vi "laneleftright413.vi"() -> ()   [LabVIEW 2015]
uses:
  <vilib>/Analysis/1siggen.llb/Ramp Pattern by Samples.vi
  G_SEN.vi
  <vilib>/Analysis/1siggen.llb/Ramp Pattern by Delta.vi
  G_ALL.vi
  G_LCM.vi
  <vilib>/Analysis/polynomials.llb/1D Polynomial Evaluation (DBL).vi
  <vilib>/Analysis/NI_AALBase.lvlib
  <vilib>/Analysis/NI_AALPro.lvlib
panel:
  out "lnum":dbl format="%.2f"
  out "rnum":dbl format="%.2f"
  out "Waveform Graph 2":dbl[](graph)
  out "w0":dbl[](array[numeric])
  out "y0":dbl[](array[numeric])
  out "x0":dbl[](array[numeric])
  out "Waveform Graph":dbl[](graph)
  out "Coeff left":dbl[](array[numeric])
  in  "iter":i32
  out "Coeff right":dbl[](array[numeric])
  out "XY Graph 4":cluster{"Y":dbl[], "Y":dbl[]}[](graph)=[{"Y"=array[3210 elements], "Y"=array[3210 elements]}, {"Y"=[-0.0, 0.001154394197769193, 0.004617650635850623, 0.010389990872226917, 0.018471784248973222, 0.02886354801042046, 0.041565947468740205, 0.056579796217107514, 0.0739060563904701, 0.0935458389742223, 0.11550040416098284, 0.13977116175580306, 0.16635967162997645, 0.19526764422393228, 0.2264969410994837, 0.26004957554195585, 0.2959277132125635, 0.3341336728515216, 0.374669927032528, 0.417539102969144, 0.4627439833735707, 0.5102875073687159, 0.560172771454063, 0.6124030305261954, 0.6669816989546717, 0.7239123517142048, 0.7831987255740245, 0.8448447203451934, 0.9088544001870815, 0.975231994973953, 1.0439819017227023, 1.1151086860829622, 1.1886170838907617, 1.2645120027869723, 1.342798523901962, 1.42348190360768, 1.5065675753387922, 1.592061151484188, 1.6799684253507792, 1.770295373200753, 1.8630481563645134, 1.9582331234307588, 2.0558568125157564, 2.1559259536137603, 2.258447471030621], "Y"=[0.0, 0.5, 1.0, 1.5, 2.0, 2.5, 3.0, 3.5, 4.0, 4.5, 5.0, 5.5, 6.0, 6.5, 7.0, 7.5, 8.0, 8.5, 9.0, 9.5, 10.0, 10.5, 11.0, 11.5, 12.0, 12.5, 13.0, 13.5, 14.0, 14.5, 15.0, 15.5, 16.0, 16.5, 17.0, 17.5, 18.0, 18.5, 19.0, 19.5, 20.0, 20.5, 21.0, 21.5, 22.0]}, {"Y"=[0.362252581831572], "Y"=[-0.8199241909738847]}, {"Y"=array[210 elements], "Y"=array[210 elements]}, {"Y"=[-0.925, -0.925, -0.925, -0.6775, -0.6775, -0.925, -0.925, -0.925, -0.925, -0.6775, -0.6775, -0.925, -0.925, -0.925, 0.9025, 0.9025, 0.9025, 0.6775, 0.6775, 0.9025, 0.9025, 0.9025, 0.9025, 0.6775, 0.6775, 0.9025, 0.9025, 0.9025, -0.925], "Y"=[-0.75, -0.224, 0.224, 0.224, -0.224, -0.224, 0.224, 2.415, 2.885, 2.885, 2.415, 2.415, 2.885, 3.5, 3.5, 2.885, 2.415, 2.415, 2.885, 2.885, 2.415, 0.224, -0.224, -0.224, 0.224, 0.224, -0.224, -0.75, -0.75]}, {"Y"=[0.171875, 0.15377271904051304, 0.1346290179491043, 0.11445423440635205, 0.09325870609283447, 0.07105277068912982, 0.04784676587581635, 0.02365102933347224, -0.0015241012573242174, -0.02766828821599482, -0.05477119386196136, -0.08282248051464558, -0.11181181049346922, -0.14172884611785413, -0.17256324970722198, -0.20430468358099463, -0.23694281005859374, -0.27046729145944115, -0.30486779010295867, -0.340133968308568, -0.3762554883956909, -0.41322201268374914, -0.4510232034921646, -0.4896487231403589], "Y"=[0.0, 0.5, 1.0, 1.5, 2.0, 2.5, 3.0, 3.5, 4.0, 4.5, 5.0, 5.5, 6.0, 6.5, 7.0, 7.5, 8.0, 8.5, 9.0, 9.5, 10.0, 10.5, 11.0, 11.5]}, {"Y"=[1.796875, 1.778772719040513, 1.7596290179491043, 1.739454234406352, 1.7182587060928345, 1.6960527706891297, 1.6728467658758164, 1.6486510293334722, 1.6234758987426758, 1.5973317117840051, 1.5702288061380387, 1.5421775194853544, 1.513188189506531, 1.483271153882146, 1.452436750292778, 1.4206953164190055, 1.3880571899414063, 1.354532708540559, 1.3201322098970414, 1.284866031691432, 1.248744511604309, 1.2117779873162509, 1.1739767965078354, 1.135351276859641, 1.0959117660522462, 1.0556686017662287, 1.014632121682167, 0.9728126634806396, 0.9302205648422242, 0.8868661634474992], "Y"=[0.0, 0.5, 1.0, 1.5, 2.0, 2.5, 3.0, 3.5, 4.0, 4.5, 5.0, 5.5, 6.0, 6.5, 7.0, 7.5, 8.0, 8.5, 9.0, 9.5, 10.0, 10.5, 11.0, 11.5, 12.0, 12.5, 13.0, 13.5, 14.0, 14.5]}, {"Y"=[-1.453125, -1.471227280959487, -1.4903709820508957, -1.510545765593648, -1.5317412939071655, -1.5539472293108703, -1.5771532341241836, -1.6013489706665278, -1.6265241012573242, -1.6526682882159949, -1.6797711938619613, -1.7078224805146456, -1.736811810493469, -1.766728846117854, -1.797563249707222, -1.8293046835809945, -1.8619428100585937, -1.895467291459441, -1.9298677901029586], "Y"=[0.0, 0.5, 1.0, 1.5, 2.0, 2.5, 3.0, 3.5, 4.0, 4.5, 5.0, 5.5, 6.0, 6.5, 7.0, 7.5, 8.0, 8.5, 9.0]}, {"Y"=[0.171875, 0.2568230007600336, 0.3384052130063493, 0.44574342526006827, 0.5205081969556753, 0.5917680690742042, 0.659409530134929, 0.7229937549325056, 0.7835496148685115, 0.8405449546633443, 0.9258576868463875], "Y"=[-20.239964538708662, -19.725637940364884, -19.211158961966362, -18.6998967366845, -18.19022720070031, -17.681887266143153, -17.17615515566314, -16.67683575591291, -16.176265245349786, -15.679082775270938, -15.183754484614711]}, {"Y"=[7.134647485270904], "Y"=[38.71960961082238]}, {"Y"=array[980 elements], "Y"=array[980 elements]}, {"Y"=[], "Y"=[]}]
  out "w":dbl[](array[numeric])
  out "y":dbl[](array[numeric])
  out "x":dbl[](array[numeric])
  out "gap":dbl
  out "rin":dbl[](array[numeric])
  out "rout":dbl[](array[numeric])
  out "r":dbl[](array[numeric])
  out "wgain":dbl[](array[numeric])
  out "y_end":dbl[](array[numeric])=[0.8601491478953653, 0.8717844136967624, 0.882947592858927, 0.8936326403234123, 0.9038337699485205, 0.9135454576426009, 0.9227624443554423, 0.9314797389261423, 0.9396926207859084, 0.9473966425143293, 0.9545876322477319, 0.9612616959383189, 0.9674152194628639, 0.9730448705798238, 0.9781476007338057, 0.9827206467064133, 0.9867615321125792, 0.9902680687415704, 0.993238357741943, 0.9956707906498045, 0.9975640502598242, 0.9989171113385246, 0.9997292411794617, 1.0, 0.9997292411794617, 0.9989171113385246, 0.9975640502598242, 0.9956707906498045, 0.993238357741943, 0.9902680687415704, 0.9867615321125792, 0.9827206467064133]
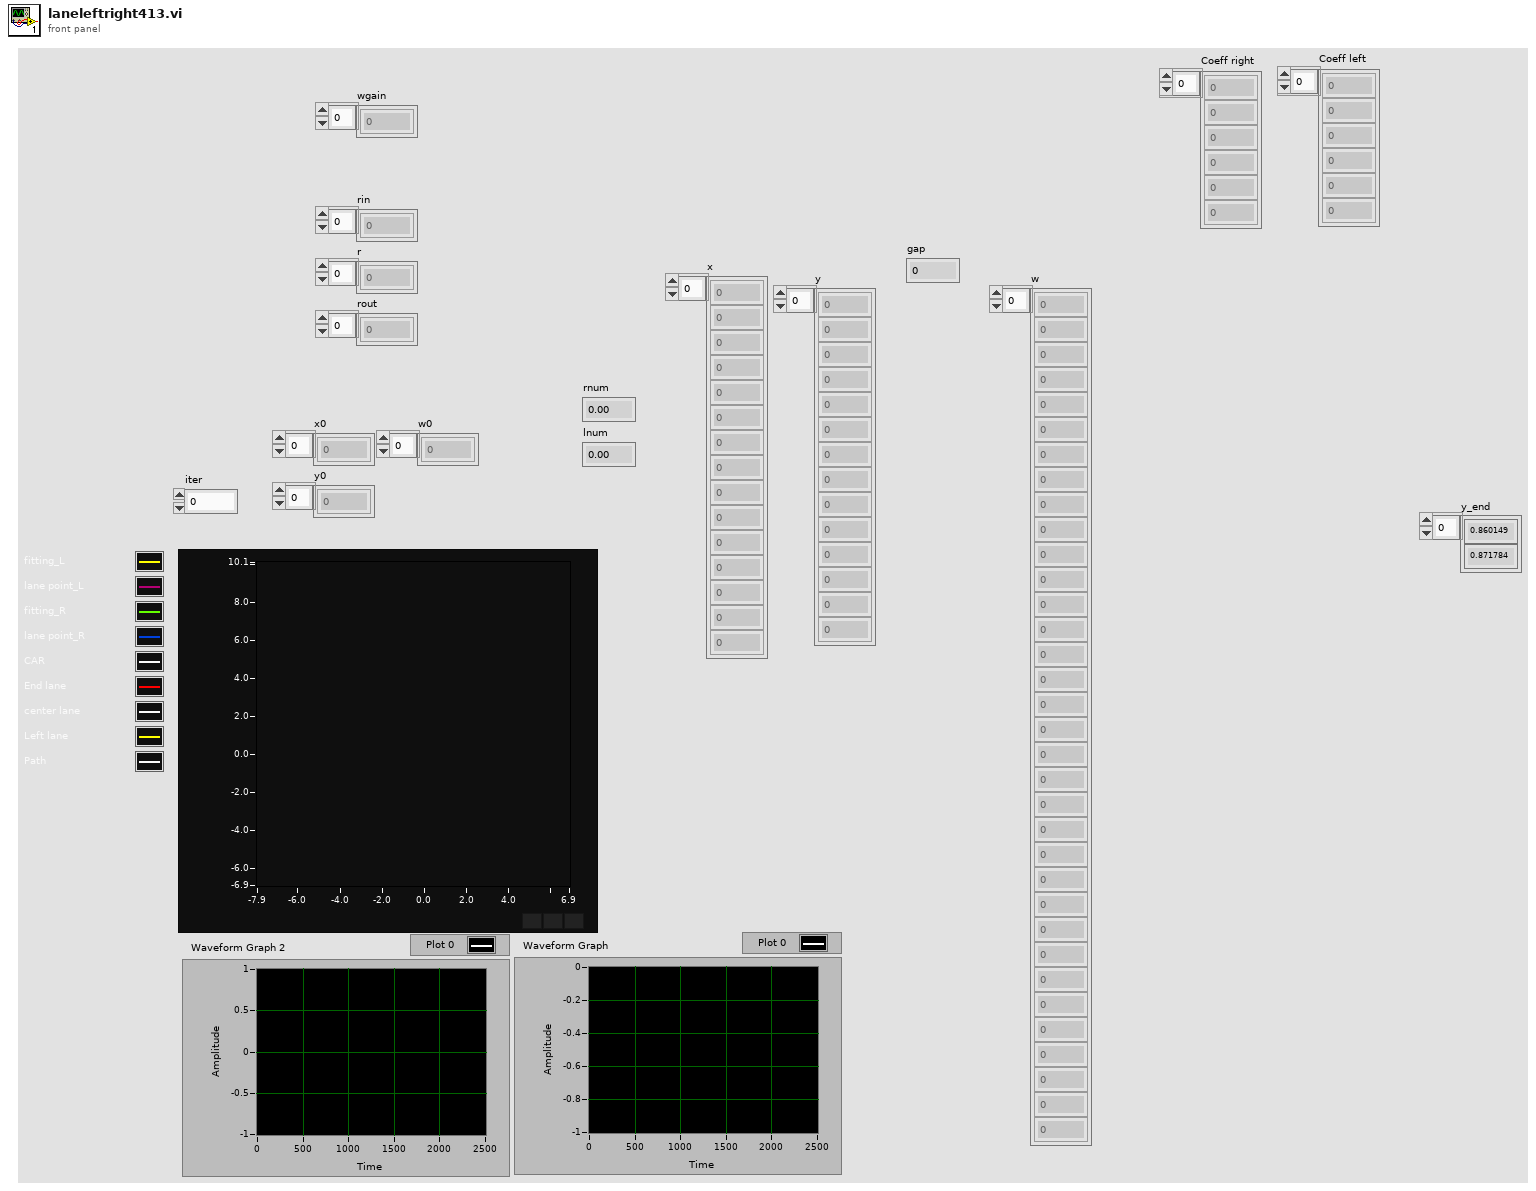
[diagram p1: front panel]
types:
  T1 = cluster{"C_Wheel base":dbl, "ratio_steer":dbl, "Overall width":dbl, "af":dbl, "turn radius":dbl, "eval":dbl, "ap":dbl, "an":dbl, "Vmax":dbl, "mu":dbl, "Vlast":dbl}
  T2 = cluster{"hash":i64, "sys time":i64, "size":i64, "x":dbl[], "y":dbl[], "point_flag":i32[]}
  T3 = cluster{"Numeric":bool, "Numeric":i32, "Rotational position":dbl, "Rotational position":dbl}[]
  T4 = cluster{bool, "Rotational position":dbl, "Rotational position":dbl}[]
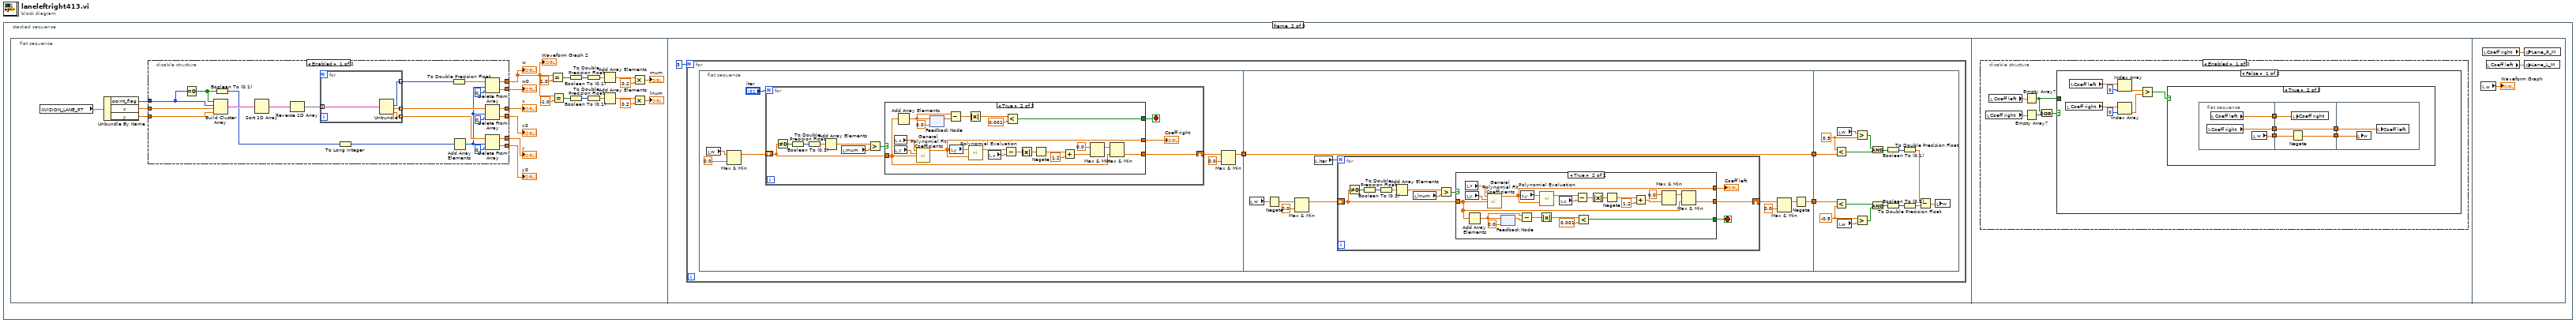
[diagram p0: block diagram]
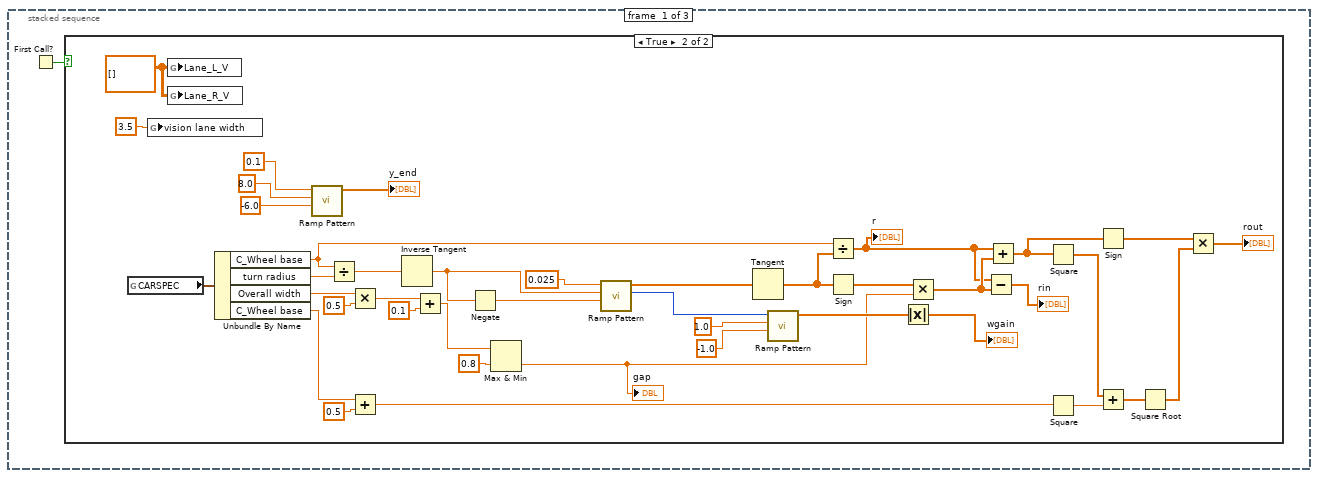
[diagram p2: hidden frame]
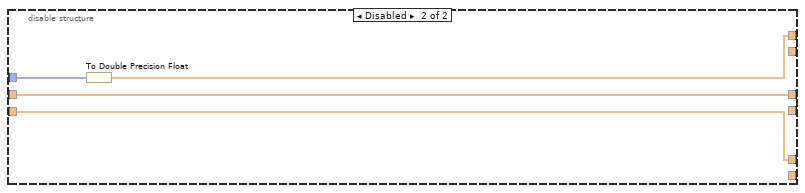
[diagram p4: hidden frame]
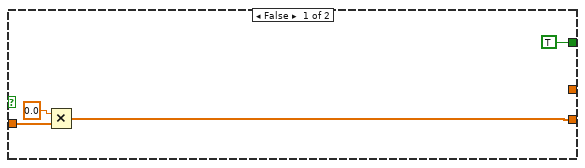
[diagram p5: hidden frame]
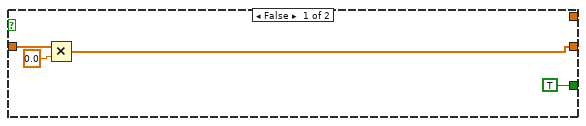
[diagram p6: hidden frame]
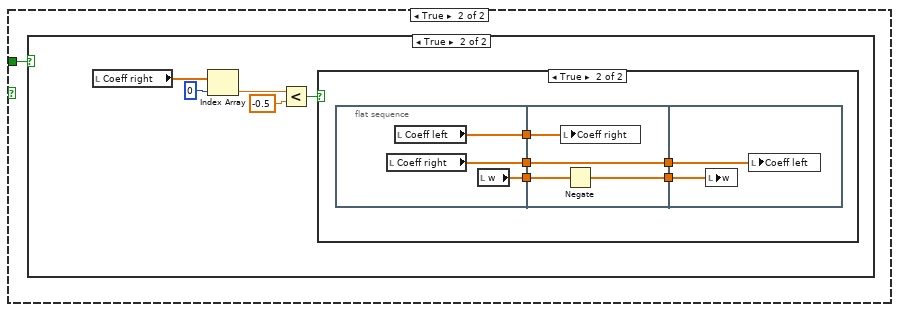
[diagram p8: hidden frame]
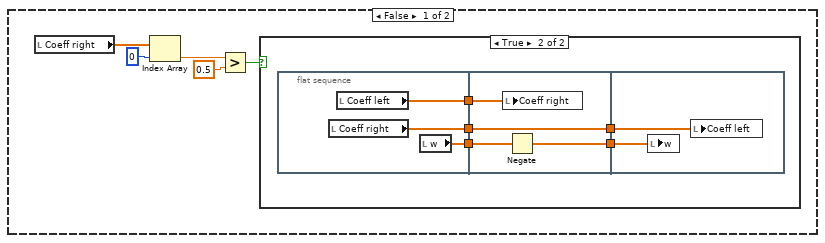
[diagram p9: hidden frame]
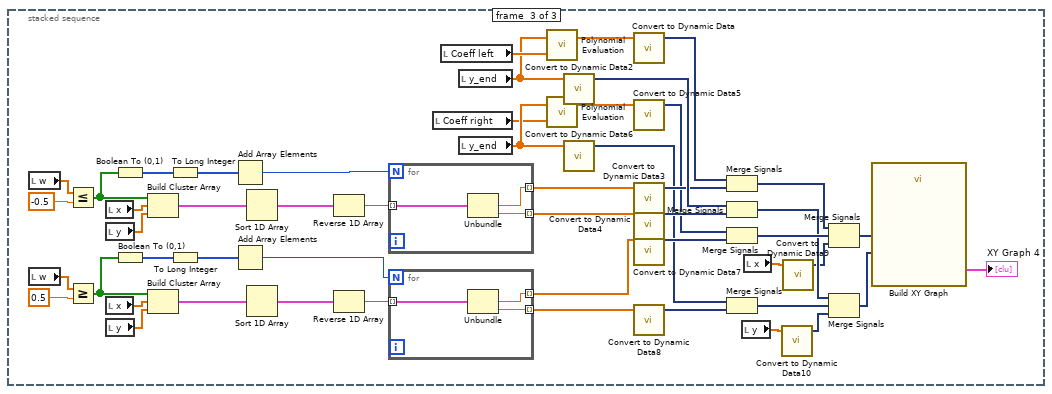
[diagram p13: hidden frame]
diagram:
  n1 = stacked-sequence {
    frame #0 {
      n2 = First Call?() -> (First Call?: T/F=w1:bool)
      n3 = case shown="True" w1 {
        frame False {
        }
        frame True {
          w37 = dbl[][] [] ("Lane_R_V")
          n4 = global read "G_ALL.vi" "CARSPEC"() -> (w10:T1)
          n5 = global write "G_SEN.vi" "vision lane width"(3.5 ("vision lane width")) -> ()
          n6 = global write "G_SEN.vi" "Lane_L_V"(w37) -> ()
          n7 = global write "G_SEN.vi" "Lane_R_V"(w37) -> ()
          n8 = Unbundle By Name(w10) -> ("C_Wheel base"=w17:dbl, "turn radius"=w11:dbl, "Overall width"=w18:dbl, "C_Wheel base"=w3:dbl)
          n9 = call-poly <vilib>:"Ramp Pattern.vi"("start"=-6.0, "end"=8.0, "delta"=0.1) -> ("Ramp Pattern"=→"y_end":dbl[])  [unwired: 6 in, 2 out]
          n10 = Divide(x=w17, y=w11) -> (x/y=w12:dbl)
          n11 = Multiply(x=w18, y=0.5) -> (x*y=w9:dbl)
          n12 = Add(x=w3, y=0.5) -> (x+y=w2:dbl)
          n13 = Inverse Tangent(1:w12) -> (0:w14:dbl)
          n14 = Add(x=w9, y=0.1) -> (x+y=w6:dbl)
          n15 = Negate(x=w14) -> (-x=w13:dbl)
          n16 = Max & Min(x=w6, y=0.8) -> (min(x,y)=w5:dbl)  [unwired: 1 out]
          "gap" <- w5
          n17 = call-poly <vilib>:"Ramp Pattern.vi"("start"=w13, "end"=w14, "delta"=0.025) -> ("samples"=w32:i32, "Ramp Pattern"=w16:dbl[])  [unwired: 6 in, 1 out]
          n18 = Tangent(1:w16) -> (0:w20:dbl[])
          n19 = call-poly <vilib>:"Ramp Pattern.vi"("start"=-1.0, "end"=1.0, "samples"=w32) -> ("Ramp Pattern"=w35:dbl[])  [unwired: 7 in, 1 out]
          n20 = Divide(x=w17, y=w20) -> (x/y=w23:dbl[])
          "r" <- w23
          n21 = Sign(1:w20) -> (0:w21:dbl[])
          n22 = Absolute Value(x=w35) -> (abs(x)=→"wgain":dbl[])
          n23 = Multiply(x=w21, y=w5) -> (x*y=w24:dbl[])
          n24 = Subtract(x=w23, y=w24) -> (x-y=→"rin":dbl[])
          n25 = Add(x=w23, y=w24) -> (x+y=w28:dbl[])
          n26 = Square(x=w28) -> (x^2=w25:dbl[])
          n27 = Square(x=w2) -> (x^2=w26:dbl)
          n28 = Sign(1:w28) -> (0:w30:dbl[])
          n29 = Add(x=w25, y=w26) -> (x+y=w27:dbl[])
          n30 = Square Root(x=w27) -> (sqrt(x)=w29:dbl[])
          n31 = Multiply(x=w30, y=w29) -> (x*y=→"rout":dbl[])
        }
      }
    }
    frame #1 {
      n32 = flat-sequence {
        frame #0 {
          n33 = global read "G_LCM.vi" "VISION_LANE_PT"() -> (w66:T2)
          n34 = Unbundle By Name(w66) -> ("point_flag"=w58:i32[], "x"=w65:dbl[], "y"=w64:dbl[])
          n35 = disable-structure shown="Enabled" {
            disable-tunnel: w58 -> [w67 w94]
            disable-tunnel: w65 -> [w68 w95]
            disable-tunnel: w64 -> [w69 w96]
            disable-tunnel: [w81 _] -> w63
            disable-tunnel: [w80 w95] -> w62
            disable-tunnel: [w77 _] -> w61
            disable-tunnel: [w76 w96] -> w60
            disable-tunnel: [w71 _] -> w59
            disable-tunnel: [w70 w97] -> w49
            frame Enabled {
              n36 = Equal To 0?(x=w67) -> (x = 0?=w84:bool[])
              n37 = Build Cluster Array(w84, w67, w68, w69) -> (w89:T3)
              n38 = Boolean To (0,1)(Boolean=w84) -> (0, 1=w83:i16[])
              n39 = Sort 1D Array(array=w89) -> (sorted array=w87:T3)
              n40 = Reverse 1D Array(array=w87) -> (reversed array=w86:T3)
              n41 = for {
                tunnel: w86 -> [w93] mode=indexing
                tunnel: [w92] -> w88 mode=indexing
                tunnel: [w91] -> w78 mode=indexing
                tunnel: [w90] -> w73 mode=indexing
                n42 = Unbundle(w93) -> ("Numeric"=w90:i32, "Rotational position"=w92:dbl, "Rotational position"=w91:dbl)  [unwired: 1 out]
              }
              n43 = To Long Integer(number=w83) -> (32bit integer=w82:i32[])
              n44 = To Double Precision Float(number=w73) -> (double precision float=w72:dbl[])
              n45 = Add Array Elements(numeric array=w82) -> (sum=w74:i32)
              n46 = Delete From Array(array=w72, length=w74, index=0) -> (deleted portion=w71:dbl[], array with subset deleted=w70:dbl[])
              n47 = Delete From Array(array=w88, length=w74, index=0) -> (deleted portion=w81:dbl[], array with subset deleted=w80:dbl[])
              n48 = Delete From Array(array=w78, length=w74, index=0) -> (deleted portion=w77:dbl[], array with subset deleted=w76:dbl[])
            }
            frame Disabled {
              n49 = To Double Precision Float(number=w94) -> (double precision float=w97:dbl[])
            }
          }
          "x" <- w62
          "y" <- w60
          "w" <- w49
          "x0" <- w63
          "y0" <- w61
          "w0" <- w59
          "Waveform Graph 2" <- w49
          n50 = Equal?(x=w49, y=1.0) -> (x = y?=w54:bool[])
          n51 = Equal?(x=w49, y=-1.0) -> (x = y?=w53:bool[])
          n52 = Boolean To (0,1)(Boolean=w54) -> (0, 1=w56:i16[])
          n53 = Boolean To (0,1)(Boolean=w53) -> (0, 1=w51:i16[])
          n54 = To Double Precision Float(number=w56) -> (double precision float=w55:dbl[])
          n55 = To Double Precision Float(number=w51) -> (double precision float=w52:dbl[])
          n56 = Add Array Elements(numeric array=w55) -> (sum=w48:dbl)
          n57 = Add Array Elements(numeric array=w52) -> (sum=w44:dbl)
          n58 = Multiply(x=w48, y=0.2) -> (x*y=→"rnum":dbl)
          n59 = Multiply(x=w44, y=0.2) -> (x*y=→"lnum":dbl)
        }
        frame #1 {
          n60 = for {
            N: 3 -> [_]
            n61 = flat-sequence {
              tunnel: [w105] -> w100
              tunnel: [w149] -> w101
              tunnel: w100 -> [w149]
              tunnel: [w148] -> w99
              tunnel: w101 -> [w202]
              tunnel: w99 -> [w198]
              frame #0 {
                n62 = local read "w"() -> (w103:dbl[])
                n63 = Max & Min(x=w103, y=0.0) -> (max(x,y)=w102:dbl[])  [unwired: 1 out]
                n64 = for {
                  N: "iter" -> [_]
                  shift-right: [w116] -> w108
                  shift-left: w102 -> [w115]
                  stop <- w118 stop-if-true
                  n65 = Not Equal To 0?(x=w115) -> (x != 0?=w114:bool[])
                  n66 = Boolean To (0,1)(Boolean=w114) -> (0, 1=w113:i16[])
                  n67 = To Double Precision Float(number=w113) -> (double precision float=w112:dbl[])
                  n68 = Add Array Elements(numeric array=w112) -> (sum=w111:dbl)
                  n69 = local read "rnum"() -> (w109:dbl)
                  n70 = Greater?(x=w111, y=w109) -> (0:w110:bool)
                  n71 = case shown="True" w110 {
                    tunnel: [TRUE w129] -> w118
                    tunnel: [_ w128] -> w117
                    tunnel: [w119 w127] -> w116
                    tunnel: w115 -> [w121 w123]
                    frame False {
                      n72 = Multiply(x=0.0, y=w121) -> (x*y=w119:dbl[])
                    }
                    frame True {
                      n73 = local read "x"() -> (w144:dbl[])
                      n74 = local read "y"() -> (w143:dbl[])
                      n75 = Add Array Elements(numeric array=w123) -> (sum=w134:dbl)
                      n76 = call <vilib>:"General Polynomial Fit Coefficients.vi"("Y"=w144, "X"=w143, "Weight"=w123) -> ("Polynomial Coefficients"=w128:dbl[])  [unwired: 11 in, 1 out]
                      n77 = feedback #1(0.0) -> (w135:dbl)
                      n78 = feedback-in #1(w134) -> ()
                      n79 = Subtract(x=w134, y=w135) -> (x-y=w132:dbl)
                      n80 = local read "y"() -> (w136:dbl[])
                      n81 = Absolute Value(x=w132) -> (abs(x)=w131:dbl)
                      n82 = call-poly <vilib>:"Polynomial Evaluation.vi"("P(x)"=w128, "A"=w136) -> ("P(A)"=w137:dbl[])  [unwired: 1 out]
                      n83 = local read "x"() -> (w138:dbl[])
                      n84 = Subtract(x=w137, y=w138) -> (x-y=w139:dbl[])
                      n85 = Less?(x=w131, y=0.001) -> (x < y?=w129:bool)
                      n86 = Absolute Value(x=w139) -> (abs(x)=w140:dbl[])
                      n87 = Negate(x=w140) -> (-x=w141:dbl[])
                      n88 = Add(x=w141, y=1.2) -> (x+y=w126:dbl[])
                      n89 = Max & Min(x=0.0, y=w126) -> (max(x,y)=w124:dbl[])  [unwired: 1 out]
                      n90 = Max & Min(x=w124, y=w123) -> (min(x,y)=w127:dbl[])  [unwired: 1 out]
                    }
                  }
                  "Coeff right" <- w117
                }
                n91 = Max & Min(x=w108, y=0.0) -> (max(x,y)=w105:dbl[])  [unwired: 1 out]
              }
              frame #1 {
                n92 = local read "w"() -> (w151:dbl[])
                n93 = Negate(x=w151) -> (-x=w146:dbl[])
                n94 = Max & Min(x=w146, y=0.0) -> (max(x,y)=w145:dbl[])  [unwired: 1 out]
                n95 = local read "iter"() -> (w150:i32)
                n96 = for {
                  N: w150 -> [_]
                  shift-right: [w162] -> w153
                  shift-left: w145 -> [w157]
                  stop <- w163 stop-if-true
                  n97 = Not Equal To 0?(x=w157) -> (x != 0?=w158:bool[])
                  n98 = Boolean To (0,1)(Boolean=w158) -> (0, 1=w159:i16[])
                  n99 = To Double Precision Float(number=w159) -> (double precision float=w160:dbl[])
                  n100 = Add Array Elements(numeric array=w160) -> (sum=w161:dbl)
                  n101 = local read "lnum"() -> (w155:dbl)
                  n102 = Greater?(x=w161, y=w155) -> (0:w156:bool)
                  n103 = case shown="True" w156 {
                    tunnel: [_ w181] -> w164
                    tunnel: [TRUE w174] -> w163
                    tunnel: w157 -> [w167 w170]
                    tunnel: [w166 w169] -> w162
                    frame False {
                      n104 = Multiply(x=w167, y=0.0) -> (x*y=w166:dbl[])
                    }
                    frame True {
                      n105 = local read "x"() -> (w190:dbl[])
                      n106 = local read "y"() -> (w189:dbl[])
                      n107 = Add Array Elements(numeric array=w170) -> (sum=w179:dbl)
                      n108 = call <vilib>:"General Polynomial Fit Coefficients.vi"("Y"=w190, "X"=w189, "Weight"=w170) -> ("Polynomial Coefficients"=w181:dbl[])  [unwired: 11 in, 1 out]
                      n109 = feedback #2(0.0) -> (w180:dbl)
                      n110 = feedback-in #2(w179) -> ()
                      n111 = Subtract(x=w179, y=w180) -> (x-y=w177:dbl)
                      n112 = local read "y"() -> (w182:dbl[])
                      n113 = Absolute Value(x=w177) -> (abs(x)=w176:dbl)
                      n114 = call-poly <vilib>:"Polynomial Evaluation.vi"("P(x)"=w181, "A"=w182) -> ("P(A)"=w183:dbl[])  [unwired: 1 out]
                      n115 = local read "x"() -> (w184:dbl[])
                      n116 = Subtract(x=w183, y=w184) -> (x-y=w185:dbl[])
                      n117 = Less?(x=w176, y=0.001) -> (x < y?=w174:bool)
                      n118 = Absolute Value(x=w185) -> (abs(x)=w186:dbl[])
                      n119 = Negate(x=w186) -> (-x=w187:dbl[])
                      n120 = Add(x=w187, y=1.2) -> (x+y=w171:dbl[])
                      n121 = Max & Min(x=0.0, y=w171) -> (max(x,y)=w173:dbl[])  [unwired: 1 out]
                      n122 = Max & Min(x=w173, y=w170) -> (min(x,y)=w169:dbl[])  [unwired: 1 out]
                    }
                  }
                  "Coeff left" <- w164
                }
                n123 = Max & Min(x=w153, y=0.0) -> (max(x,y)=w154:dbl[])  [unwired: 1 out]
                n124 = Negate(x=w154) -> (-x=w148:dbl[])
              }
              frame #2 {
                w199 = -0.5
                w201 = 0.5
                n125 = Less?(x=w201, y=w202) -> (x < y?=w205:bool[])
                n126 = Less?(x=w198, y=w199) -> (x < y?=w203:bool[])
                n127 = local read "w"() -> (w207:dbl[])
                n128 = local read "w"() -> (w200:dbl[])
                n129 = Greater?(x=w207, y=w201) -> (0:w206:bool[])
                n130 = Greater?(x=w199, y=w200) -> (0:w204:bool[])
                n131 = And(x=w206, y=w205) -> (x .and. y?=w196:bool[])
                n132 = And(x=w203, y=w204) -> (x .and. y?=w194:bool[])
                n133 = Boolean To (0,1)(Boolean=w196) -> (0, 1=w197:i16[])
                n134 = Boolean To (0,1)(Boolean=w194) -> (0, 1=w195:i16[])
                n135 = To Double Precision Float(number=w197) -> (double precision float=w193:dbl[])
                n136 = To Double Precision Float(number=w195) -> (double precision float=w192:dbl[])
                n137 = Subtract(x=w193, y=w192) -> (x-y=w191:dbl[])
                n138 = local write "w"(w191) -> ()
              }
            }
          }
        }
        frame #2 {
          n139 = disable-structure shown="Enabled" {
            frame Enabled {
              n140 = local read "Coeff right"() -> (w211:dbl[])
              n141 = local read "Coeff left"() -> (w212:dbl[])
              n142 = Empty Array?(array=w212) -> (empty?=w208:bool)
              n143 = Empty Array?(array=w211) -> (empty?=w210:bool)
              n144 = Exclusive Or(1:w210, 2:w208) -> (0:w209:bool)
              n145 = case shown="False" w209 {
                tunnel: w208 -> [_ w234]
                frame False {
                  n146 = local read "Coeff right"() -> (w216:dbl[])
                  n147 = local read "Coeff left"() -> (w219:dbl[])
                  n148 = Index Array(array=w219, index=0) -> (element=w215:dbl)
                  n149 = Index Array(array=w216, index=0) -> (element=w214:dbl)
                  n150 = Greater?(x=w215, y=w214) -> (0:w213:bool)
                  n151 = case shown="True" w213 {
                    frame False {
                    }
                    frame True {
                      n152 = flat-sequence {
                        tunnel: [w227] -> w224
                        tunnel: [w226] -> w223
                        tunnel: [w225] -> w221
                        tunnel: w224 -> [w231]
                        tunnel: w223 -> [w230]
                        tunnel: [w230] -> w222
                        tunnel: w221 -> [w229]
                        tunnel: [w228] -> w220
                        tunnel: w222 -> [w233]
                        tunnel: w220 -> [w232]
                        frame #0 {
                          n153 = local read "Coeff right"() -> (w226:dbl[])
                          n154 = local read "Coeff left"() -> (w227:dbl[])
                          n155 = local read "w"() -> (w225:dbl[])
                        }
                        frame #1 {
                          n156 = Negate(x=w229) -> (-x=w228:dbl[])
                          n157 = local write "Coeff right"(w231) -> ()
                        }
                        frame #2 {
                          n158 = local write "w"(w232) -> ()
                          n159 = local write "Coeff left"(w233) -> ()
                        }
                      }
                    }
                  }
                }
                frame True {
                  n160 = case shown="True" w234 {
                    frame False {
                      n161 = local read "Coeff right"() -> (w239:dbl[])
                      n162 = Index Array(array=w239, index=0) -> (element=w236:dbl)
                      n163 = Greater?(x=w236, y=0.5) -> (0:w235:bool)
                      n164 = case shown="True" w235 {
                        frame False {
                        }
                        frame True {
                          n165 = flat-sequence {
                            tunnel: [w247] -> w244
                            tunnel: [w246] -> w243
                            tunnel: [w245] -> w242
                            tunnel: w244 -> [w251]
                            tunnel: w243 -> [w250]
                            tunnel: [w250] -> w241
                            tunnel: w242 -> [w249]
                            tunnel: [w248] -> w240
                            tunnel: w241 -> [w253]
                            tunnel: w240 -> [w252]
                            frame #0 {
                              n166 = local read "Coeff right"() -> (w246:dbl[])
                              n167 = local read "Coeff left"() -> (w247:dbl[])
                              n168 = local read "w"() -> (w245:dbl[])
                            }
                            frame #1 {
                              n169 = local write "Coeff right"(w251) -> ()
                              n170 = Negate(x=w249) -> (-x=w248:dbl[])
                            }
                            frame #2 {
                              n171 = local write "w"(w252) -> ()
                              n172 = local write "Coeff left"(w253) -> ()
                            }
                          }
                        }
                      }
                    }
                    frame True {
                      n173 = local read "Coeff right"() -> (w258:dbl[])
                      n174 = Index Array(array=w258, index=0) -> (element=w255:dbl)
                      n175 = Less?(x=w255, y=-0.5) -> (x < y?=w254:bool)
                      n176 = case shown="True" w254 {
                        frame False {
                        }
                        frame True {
                          n177 = flat-sequence {
                            tunnel: [w266] -> w263
                            tunnel: [w265] -> w262
                            tunnel: [w264] -> w261
                            tunnel: w263 -> [w270]
                            tunnel: w262 -> [w269]
                            tunnel: [w269] -> w260
                            tunnel: w261 -> [w268]
                            tunnel: [w267] -> w259
                            tunnel: w260 -> [w272]
                            tunnel: w259 -> [w271]
                            frame #0 {
                              n178 = local read "Coeff right"() -> (w265:dbl[])
                              n179 = local read "Coeff left"() -> (w266:dbl[])
                              n180 = local read "w"() -> (w264:dbl[])
                            }
                            frame #1 {
                              n181 = local write "Coeff right"(w270) -> ()
                              n182 = Negate(x=w268) -> (-x=w267:dbl[])
                            }
                            frame #2 {
                              n183 = local write "w"(w271) -> ()
                              n184 = local write "Coeff left"(w272) -> ()
                            }
                          }
                        }
                      }
                    }
                  }
                }
              }
            }
            frame Disabled {
            }
          }
        }
        frame #3 {
          n185 = local read "w"() -> (→"Waveform Graph":dbl[])
          n186 = local read "Coeff right"() -> (w274:dbl[])
          n187 = local read "Coeff left"() -> (w275:dbl[])
          n188 = global write "G_SEN.vi" "Lane_R_M"(w274) -> ()
          n189 = global write "G_SEN.vi" "Lane_L_M"(w275) -> ()
        }
      }
    }
    frame #2 {
      n190 = local read "w"() -> (w320:dbl[])
      n191 = local read "w"() -> (w291:dbl[])
      n192 = Less Or Equal?(x=w320, y=-0.5) -> (x <= y?=w313:bool[])
      n193 = Greater Or Equal?(x=w291, y=0.5) -> (x >= y?=w298:bool[])
      n194 = local read "x"() -> (w316:dbl[])
      n195 = local read "y"() -> (w315:dbl[])
      n196 = local read "x"() -> (w295:dbl[])
      n197 = local read "y"() -> (w296:dbl[])
      n198 = Boolean To (0,1)(Boolean=w313) -> (0, 1=w312:i16[])
      n199 = Boolean To (0,1)(Boolean=w298) -> (0, 1=w299:i16[])
      n200 = Build Cluster Array(w313, w316, w315) -> (w317:T4)
      n201 = Build Cluster Array(w298, w295, w296) -> (w294:T4)
      n202 = To Long Integer(number=w312) -> (32bit integer=w311:i32[])
      n203 = To Long Integer(number=w299) -> (32bit integer=w300:i32[])
      n204 = Add Array Elements(numeric array=w311) -> (sum=w310:i32)
      n205 = Add Array Elements(numeric array=w300) -> (sum=w301:i32)
      n206 = Sort 1D Array(array=w317) -> (sorted array=w318:T4)
      n207 = Sort 1D Array(array=w294) -> (sorted array=w293:T4)
      n208 = Reverse 1D Array(array=w318) -> (reversed array=w314:T4)
      n209 = Reverse 1D Array(array=w293) -> (reversed array=w297:T4)
      n210 = for {
        N: w310 -> [_]
        tunnel: w314 -> [w332] mode=indexing
        tunnel: [w331] -> w309 mode=indexing
        tunnel: [w330] -> w307 mode=indexing
        n211 = Unbundle(w332) -> ("Rotational position"=w331:dbl, "Rotational position"=w330:dbl)  [unwired: 1 out]
      }
      n212 = for {
        N: w301 -> [_]
        tunnel: w297 -> [w329] mode=indexing
        tunnel: [w328] -> w302 mode=indexing
        tunnel: [w327] -> w304 mode=indexing
        n213 = Unbundle(w329) -> ("Rotational position"=w328:dbl, "Rotational position"=w327:dbl)  [unwired: 1 out]
      }
      n214 = local read "Coeff right"() -> (w286:dbl[])
      n215 = local read "Coeff left"() -> (w325:dbl[])
      n216 = local read "y_end"() -> (w322:dbl[])
      n217 = local read "y_end"() -> (w289:dbl[])
      n218 = call-poly <vilib>:"Polynomial Evaluation.vi"("P(x)"=w325, "A"=w322) -> ("P(A)"=w324:dbl[])  [unwired: 1 out]
      n219 = call-poly <vilib>:"Polynomial Evaluation.vi"("P(x)"=w286, "A"=w289) -> ("P(A)"=w287:dbl[])  [unwired: 1 out]
      n220 = call "Convert to Dynamic Data2"("Array"=w322) -> ("Dynamic Data Type"=w321:dynamicdata)  [unwired: 3 in]
      n221 = call "Convert to Dynamic Data6"("Array"=w289) -> ("Dynamic Data Type"=w290:dynamicdata)  [unwired: 3 in]
      n222 = call "Convert to Dynamic Data"("Array"=w324) -> ("Dynamic Data Type"=w323:dynamicdata)  [unwired: 3 in]
      n223 = call "Convert to Dynamic Data5"("Array"=w287) -> ("Dynamic Data Type"=w288:dynamicdata)  [unwired: 3 in]
      n224 = call "Convert to Dynamic Data3"("Array"=w309) -> ("Dynamic Data Type"=w308:dynamicdata)  [unwired: 3 in]
      n225 = call "Convert to Dynamic Data4"("Array"=w307) -> ("Dynamic Data Type"=w306:dynamicdata)  [unwired: 3 in]
      n226 = call "Convert to Dynamic Data7"("Array"=w302) -> ("Dynamic Data Type"=w303:dynamicdata)  [unwired: 3 in]
      n227 = call "Convert to Dynamic Data8"("Array"=w304) -> ("Dynamic Data Type"=w305:dynamicdata)  [unwired: 3 in]
      n228 = Merge Signals(w323, w308) -> (w285:dynamicdata)
      n229 = Merge Signals(w321, w306) -> (w282:dynamicdata)
      n230 = Merge Signals(w288, w303) -> (w284:dynamicdata)
      n231 = Merge Signals(w290, w305) -> (w281:dynamicdata)
      n232 = local read "y"() -> (w277:dbl[])
      n233 = local read "x"() -> (w279:dbl[])
      n234 = call "Convert to Dynamic Data10"("Array"=w277) -> ("Dynamic Data Type"=w276:dynamicdata)  [unwired: 3 in]
      n235 = call "Convert to Dynamic Data9"("Array"=w279) -> ("Dynamic Data Type"=w278:dynamicdata)  [unwired: 3 in]
      n236 = Merge Signals(w285, w284, w278) -> (w283:dynamicdata)
      n237 = Merge Signals(w282, w281, w276) -> (w280:dynamicdata)
      n238 = call "Build XY Graph"("Y Input"=w280, "X Input"=w283) -> ("XY Graph"=→"XY Graph 4":cluster{"X":dbl[], "Y":dbl[]}[])  [unwired: 8 in, 1 out]
    }
  }
